vi "TDT One Shot Test.vi"() -> ()   [LabVIEW 2020]
uses:
  Typedefs/TDT-Output source.ctl
  Typedefs/TDT-Device ID.ctl
  Signal Synthesis VIs/4th Generation/Classes/Level/LevelUnits.ctl
  Signal Synthesis VIs/4th Generation/Classes/SignalManager/SignalManager.lvclass/SignalManager.ctl
  Signal Synthesis VIs/4th Generation/Classes/Channel/Channel.lvclass/Channel.ctl
  6aa364f9-6b6d-4e7c-9406-0d56994a8018.vi
  Signal Synthesis VIs/4th Generation/Classes/Channel/Write Waveform.vi
  Signal Synthesis VIs/4th Generation/Classes/Channel/Write Gate.vi
  Signal Synthesis VIs/4th Generation/Classes/Channel/Write Level.vi
  Signal Synthesis VIs/4th Generation/Classes/Channel/Write Destination.vi
  Signal Synthesis VIs/4th Generation/Classes/SignalManager/Write Destinations.vi
  Signal Synthesis VIs/4th Generation/Classes/Waveforms/Tone/Tone.lvclass
  D:/Development/epl-vi-lib/Signal Synthesis VIs/4th Generation/Classes/Waveforms/Waveform/Waveform.lvclass
  Signal Synthesis VIs/4th Generation/Classes/Channel/Channel.lvclass
  Signal Synthesis VIs/4th Generation/Classes/Level/Level.lvclass
  Signal Synthesis VIs/4th Generation/Classes/Gate/Gate.lvclass
  Signal Synthesis VIs/4th Generation/Classes/SignalManager/SignalManager.lvclass
panel:
  out "ramping":bool
  out "GetTagVal":sgl
  out "Graph":dbl[][](graph)
  in  "Duration (ms)":dbl=5000.0
  in  "AO Sampling Rate (Hz)":dbl=25000.0
  in  "stop":bool
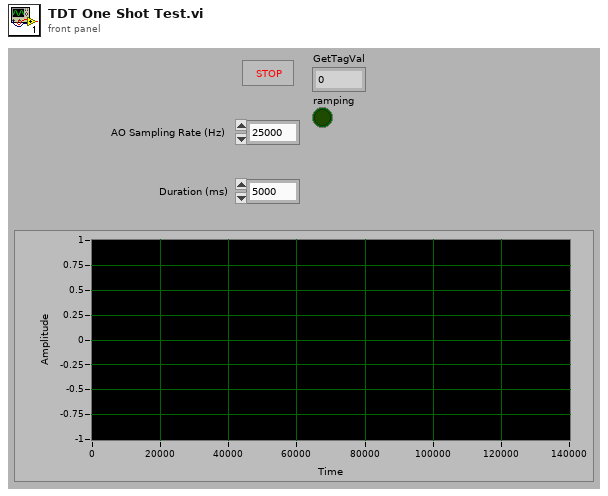
[diagram p1: front panel]
types:
  T1 = typedef "Level.lvclass/LevelUnits.ctl" = enum16{"dB atten", "dB SPL", "dB Vrms", "Volts", "dB mW", "mW", "dB HL", "dB SL"}
  T2 = typedef "TDT-Output source.ctl" = cluster{"Device":T3, "Num":i32}
  T3 = typedef "TDT-Device ID.ctl" = enum16{"None", "PA5", "RP2", "RL2", "RA16", "RV8", "RX5", "RX6", "RX7", "RX8", "RZ2", "RZ5", "RZ6"}
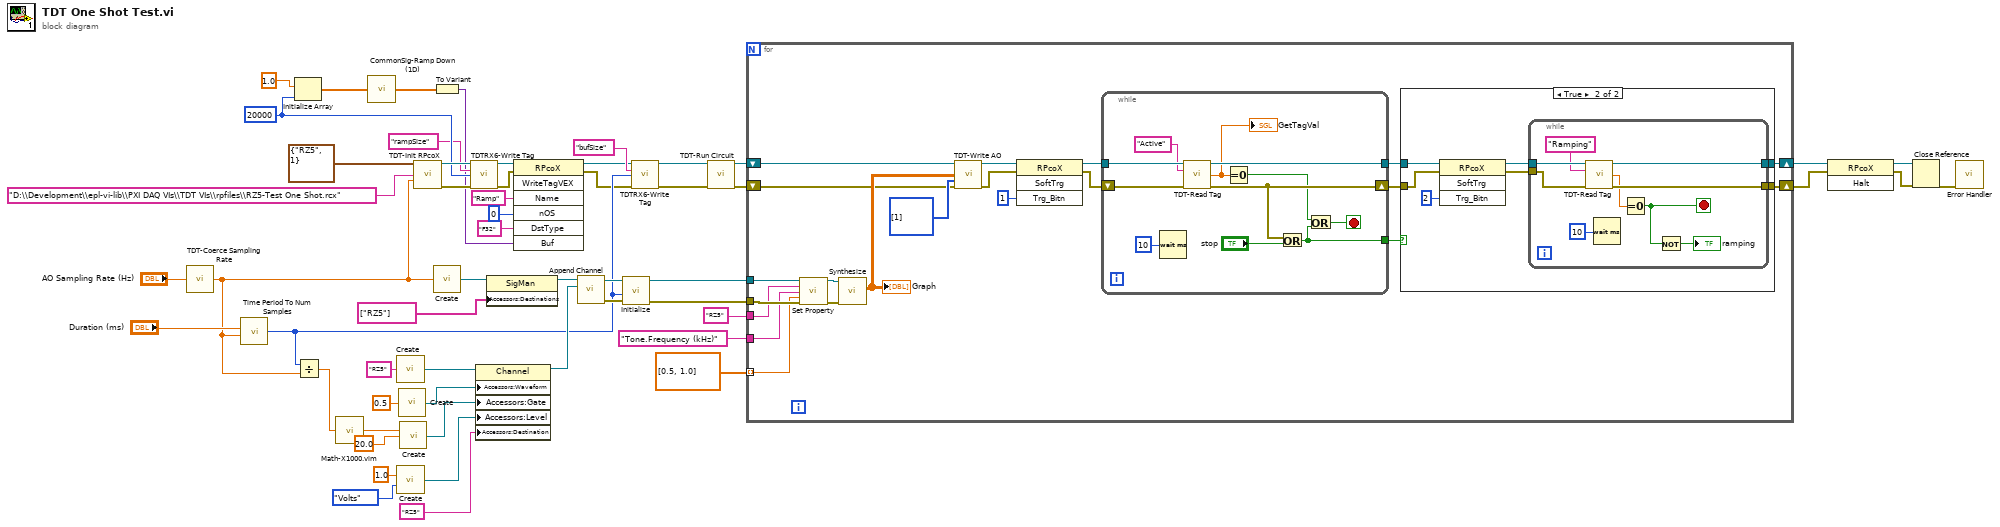
[diagram p0: block diagram]
diagram:
  w11 = 20000 ("dimension size")
  n1 = call "TDT-Coerce Sampling Rate.vi"("Fs (Hz)"="AO Sampling Rate (Hz)") -> ("Coerced"=w29:dbl)
  n2 = call "Time Period To Num Samples.vi"("Duration (ms)"="Duration (ms)", "Sampling rate (Hz)"=w29) -> ("Samples"=w24:i32)  [unwired: 5 in]
  n3 = Initialize Array(1.0, w11) -> (w14:dbl[])
  n4 = Divide(x=w24, y=w29) -> (x/y=w28:dbl)
  n5 = call "Math-X1000.vim"("X"=w28) -> ("1000X"=w27:dbl)
  n6 = call "CommonSig-Ramp Down (1D).vi"("Array"=w14) -> ("Ramped array"=w3:dbl[])  [unwired: 4 in]
  n7 = call "Create.vi"("Name"="RZ5" ("Destination")) -> ("Channel"=w44:refnum<class "Channel.lvclass">)  [unwired: 14 in]
  n8 = call "Create.vi"("Value"=1.0, "Units"=LevelUnits."Volts") -> ("Level"=w47:refnum<class "Level.lvclass">)  [unwired: 13 in]
  n9 = call "Create.vi"("Frequency (kHz)"=0.5) -> ("Tone"=w45:refnum<class "Tone.lvclass">)  [unwired: 14 in]
  n10 = call "Create.vi"("Duration (ms)"=w27, "Ramp (ms)"=20.0) -> ("Gate"=w46:refnum<class "Gate.lvclass">)  [unwired: 13 in]
  n11 = call "TDT-Init RPcoX.vi"("Output"=T2 {"Device"=enum."RZ5", "Num"=1}, "RPfilename"="D:\\Development\\epl-vi-lib\\PXI DAQ VIs\\TDT VIs\\rpfiles\\RZ5-Test One Shot.rcx", "Sampling rate (Hz)"=w29) -> ("RPcoX"=w12:refnum<k7>, "error out"=w13:errorcluster)  [unwired: 11 in]
  n12 = call "Create.vi"("Fs (Hz)"=w29) -> ("SigMan"=w39:refnum<class "SignalManager.lvclass">)  [unwired: 14 in]
  n13 = To Variant(anything=w3) -> (Variant=w2:variant)
  n14 = call "TDTRX6-Write Tag.vi"("RPcox"=w12, "Name"="rampSize", "Value"=w11, "error in"=w13) -> ("RPcox Out"=w9:refnum<k7>, "error out"=w6:errorcluster)  [unwired: 10 in]
  n15 = property class="Channel"(reference=w44, "Accessors:Waveform"=w45, "Accessors:Gate"=w46, "Accessors:Level"=w47, "Accessors:Destination"="RZ5" ("Destination")) -> (reference out=w36:refnum<class "Channel.lvclass">)  [unwired: 1 in, 1 out]
  n16 = property class="SigMan"(reference=w39, "Accessors:Destinations"=string[] ["RZ5"] ("Destination")) -> (reference out=w37:refnum<class "SignalManager.lvclass">)  [unwired: 1 in, 1 out]
  n17 = invoke class="RPcoX" method="WriteTagVEX"(reference=w9, error in=w6, "Name"="Ramp", "nOS"=0, "DstType"="F32", "Buf"=w2) -> (reference out=w8:refnum<k7>, error out=w7:errorcluster)  [unwired: 1 in, 5 out]
  n18 = call "Append Channel.vi"("Channel"=w36, "SignalManager in"=w37) -> ("error out"=w31:errorcluster, "SignalManager out"=w35:refnum<class "SignalManager.lvclass">)  [unwired: 8 in]
  n19 = call "Initialize.vi"("error in (no error)"=w31, "Npts"=w24, "SigMan in"=w35) -> ("error out"=w30:errorcluster, "SigMan out"=w32:refnum<class "SignalManager.lvclass">)  [unwired: 7 in]
  n20 = call "TDTRX6-Write Tag.vi"("RPcox"=w8, "Name"="bufSize", "Value"=w24, "error in"=w7) -> ("RPcox Out"=w23:refnum<k7>, "error out"=w22:errorcluster)  [unwired: 10 in]
  n21 = call "TDT-Run Circuit.vi"("RPcoX"=w23, "error in (no error)"=w22) -> ("RPcoX out"=w20:refnum<k7>, "error out"=w21:errorcluster)  [unwired: 12 in]
  n22 = for {
    tunnel: w32 -> [w66]
    tunnel: w30 -> [w65]
    shift-right: [w55] -> w25
    shift-left: w21 -> [w70]
    shift-right: [w56] -> w26
    shift-left: w20 -> [w69]
    tunnel: "RZ5" ("Destination") -> [w62]
    tunnel: "Tone.Frequency (kHz)" ("Destination") -> [w61]
    tunnel: dbl[] [0.5, 1.0] -> [w60] mode=indexing
    n23 = call "Set Property.vi"("SigMan in"=w66, "chan"=w62, "param"=w61, "value"=w60, "error in (no error)"=w65) -> ("SigMan out"=w64:refnum<class "SignalManager.lvclass">, "error out"=w63:errorcluster)  [unwired: 9 in]
    n24 = call "Synthesize.vi"("error in (no error)"=w63, "SigMan in"=w64) -> ("Array"=w74:dbl[][])  [unwired: 7 in, 2 out]
    "Graph" <- w74
    n25 = call "TDT-Write AO.vi"("RPcox"=w69, "Input array"=w74, "Chans"=i32[] [1], "error in (no error)"=w70) -> ("RPcox (thru)"=w68:refnum<k7>, "error out"=w67:errorcluster)  [unwired: 10 in]
    n26 = invoke class="RPcoX" method="SoftTrg"(reference=w68, error in=w67, "Trg_Bitn"=1) -> (reference out=w73:refnum<k7>, error out=w72:errorcluster)  [unwired: 1 in, 2 out]
    n27 = while {
      tunnel: w73 -> [w104]
      tunnel: [w101] -> w57
      shift-right: [w102] -> w58
      shift-left: w72 -> [w103]
      tunnel: [w95] -> w59
      stop <- w96 stop-if-true
      n28 = Wait (ms)(milliseconds to wait=u32 10) -> ()  [unwired: 1 out]
      n29 = call "TDT-Read Tag.vi"("RPcox"=w104, "Name"="Active", "error in"=w103) -> ("RPcox Out"=w101:refnum<k7>, "GetTagVal"=w98:sgl, "error out"=w102:errorcluster)  [unwired: 10 in]
      "GetTagVal" <- w98
      n30 = Equal To 0?(x=w98) -> (x = 0?=w94:bool)
      n31 = Or(x=w102, y="stop") -> (x .or. y?=w95:bool)
      n32 = Or(x=w94, y=w95) -> (x .or. y?=w96:bool)
    }
    n33 = case shown="True" w59 {
      tunnel: w58 -> [w76 w83]
      tunnel: w57 -> [w77 w84]
      tunnel: [w77 w79] -> w56
      tunnel: [w76 w78] -> w55
      frame False {
      }
      frame True {
        n34 = invoke class="RPcoX" method="SoftTrg"(reference=w84, error in=w83, "Trg_Bitn"=2) -> (reference out=w81:refnum<k7>, error out=w80:errorcluster)  [unwired: 1 in, 2 out]
        n35 = while {
          tunnel: w81 -> [w93]
          tunnel: w80 -> [w92]
          tunnel: [w91] -> w79
          tunnel: [w90] -> w78
          stop <- w87 stop-if-true
          n36 = call "TDT-Read Tag.vi"("RPcox"=w93, "Name"="Ramping", "error in"=w92) -> ("RPcox Out"=w91:refnum<k7>, "GetTagVal"=w88:sgl, "error out"=w90:errorcluster)  [unwired: 10 in]
          n37 = Wait (ms)(milliseconds to wait=u32 10) -> ()  [unwired: 1 out]
          n38 = Equal To 0?(x=w88) -> (x = 0?=w87:bool)
          n39 = Not(x=w87) -> (.not. x?=→"ramping":bool)
        }
      }
    }
  }
  n40 = invoke class="RPcoX" method="Halt"(reference=w26, error in=w25) -> (reference out=w50:refnum<k7>, error out=w49:errorcluster)  [unwired: 1 in, 1 out]
  n41 = Close Reference(reference=w50, error in (no error)=w49) -> (error out=w48:errorcluster)
  n42 = call "Error Handler.vi"("error in (no error)"=w48) -> ()  [unwired: 12 in, 3 out]
